vi "main.vi"() -> ()   [LabVIEW 2024]
panel:
  out "Column Names":string[](array[string])
  out "Result Set 3":string[][](table)
  out "?":string[](array[string])
  in  "?":bool
  in  "num_cmd 4":string
  in  "Suppression de la commande":bool
  in  "num_cmd 3":string
  in  "?":bool
  in  "num_cmd 2":string
  in  "date livraison":string
  in  "?":bool
  in  "id produit":string
  in  "nom_produit":string
  in  "date_livraison":string
  in  "date_commande":string
  in  "adresse_client":string
  in  "tele_client":string
  in  "nom_pre_client":string
  in  "status_liv":string
  in  "quantite":string
  in  "description":string
  in  "num_cmd":string
  out "?":string[][](table)
  out "?":string[](array[string])
  out "Result Set 2":string[][](table)
  out "Result Set":string[][](table)
  out "Salaire brut":dbl
  out "Salaire net":dbl
  out "Cout des salaires":dbl
  in  "button calc salaire":bool
  in  "Taux horaire":dbl
  out "notions_cles":dbl[](array[numeric])
  in  "Calculs button":bool
  in  "Impots":dbl
  in  "CA":dbl
  in  "Argent ventes":dbl
  in  "dettes":dbl
  out "Taches":string[][](table) caption="Taches salarié"
  out "Pointages":string[][](table)
  in  "OK Button":bool
  in  "Action":i16(ring) items=["Supprimer un employé", "Ajouter un employé"]
  in  "Choix":i16(ring) items=["admin", "alexis", "julien", "florian", "saco", "aaaaa"]
  in  "Projet":i16(ring) items=["Meuble"]
  out "Taches du projet":string[][](table)
  out "Identifiant de l'employé":string
  out "Code du Poste":dbl
  out "Prénom":string
  out "Nom":string
  out "?":string
  in  "Annuler Licenciement":bool
  in  "Valider Licenciement":bool
  out "?":string
  in  "Annuler Recrutement":bool
  in  "Valider Recrutement":bool
  in  "Mot de passe administrateur":string
  in  "Identifiant de l'employé":string
  in  "Supprimer l'employé":bool
  out "?":string
  in  "Licenciement":bool
  out "?":string
  out "?":string
  in  "Ajouter l'employé":bool
  in  "stop":bool
  in  "Code du Poste":dbl
  in  "Prénom":string
  in  "Nom":string
  in  "Recrutement":bool
  in  "MDP":string
  in  "ID":string
  out "État":string
  in  "Déconnexion":bool
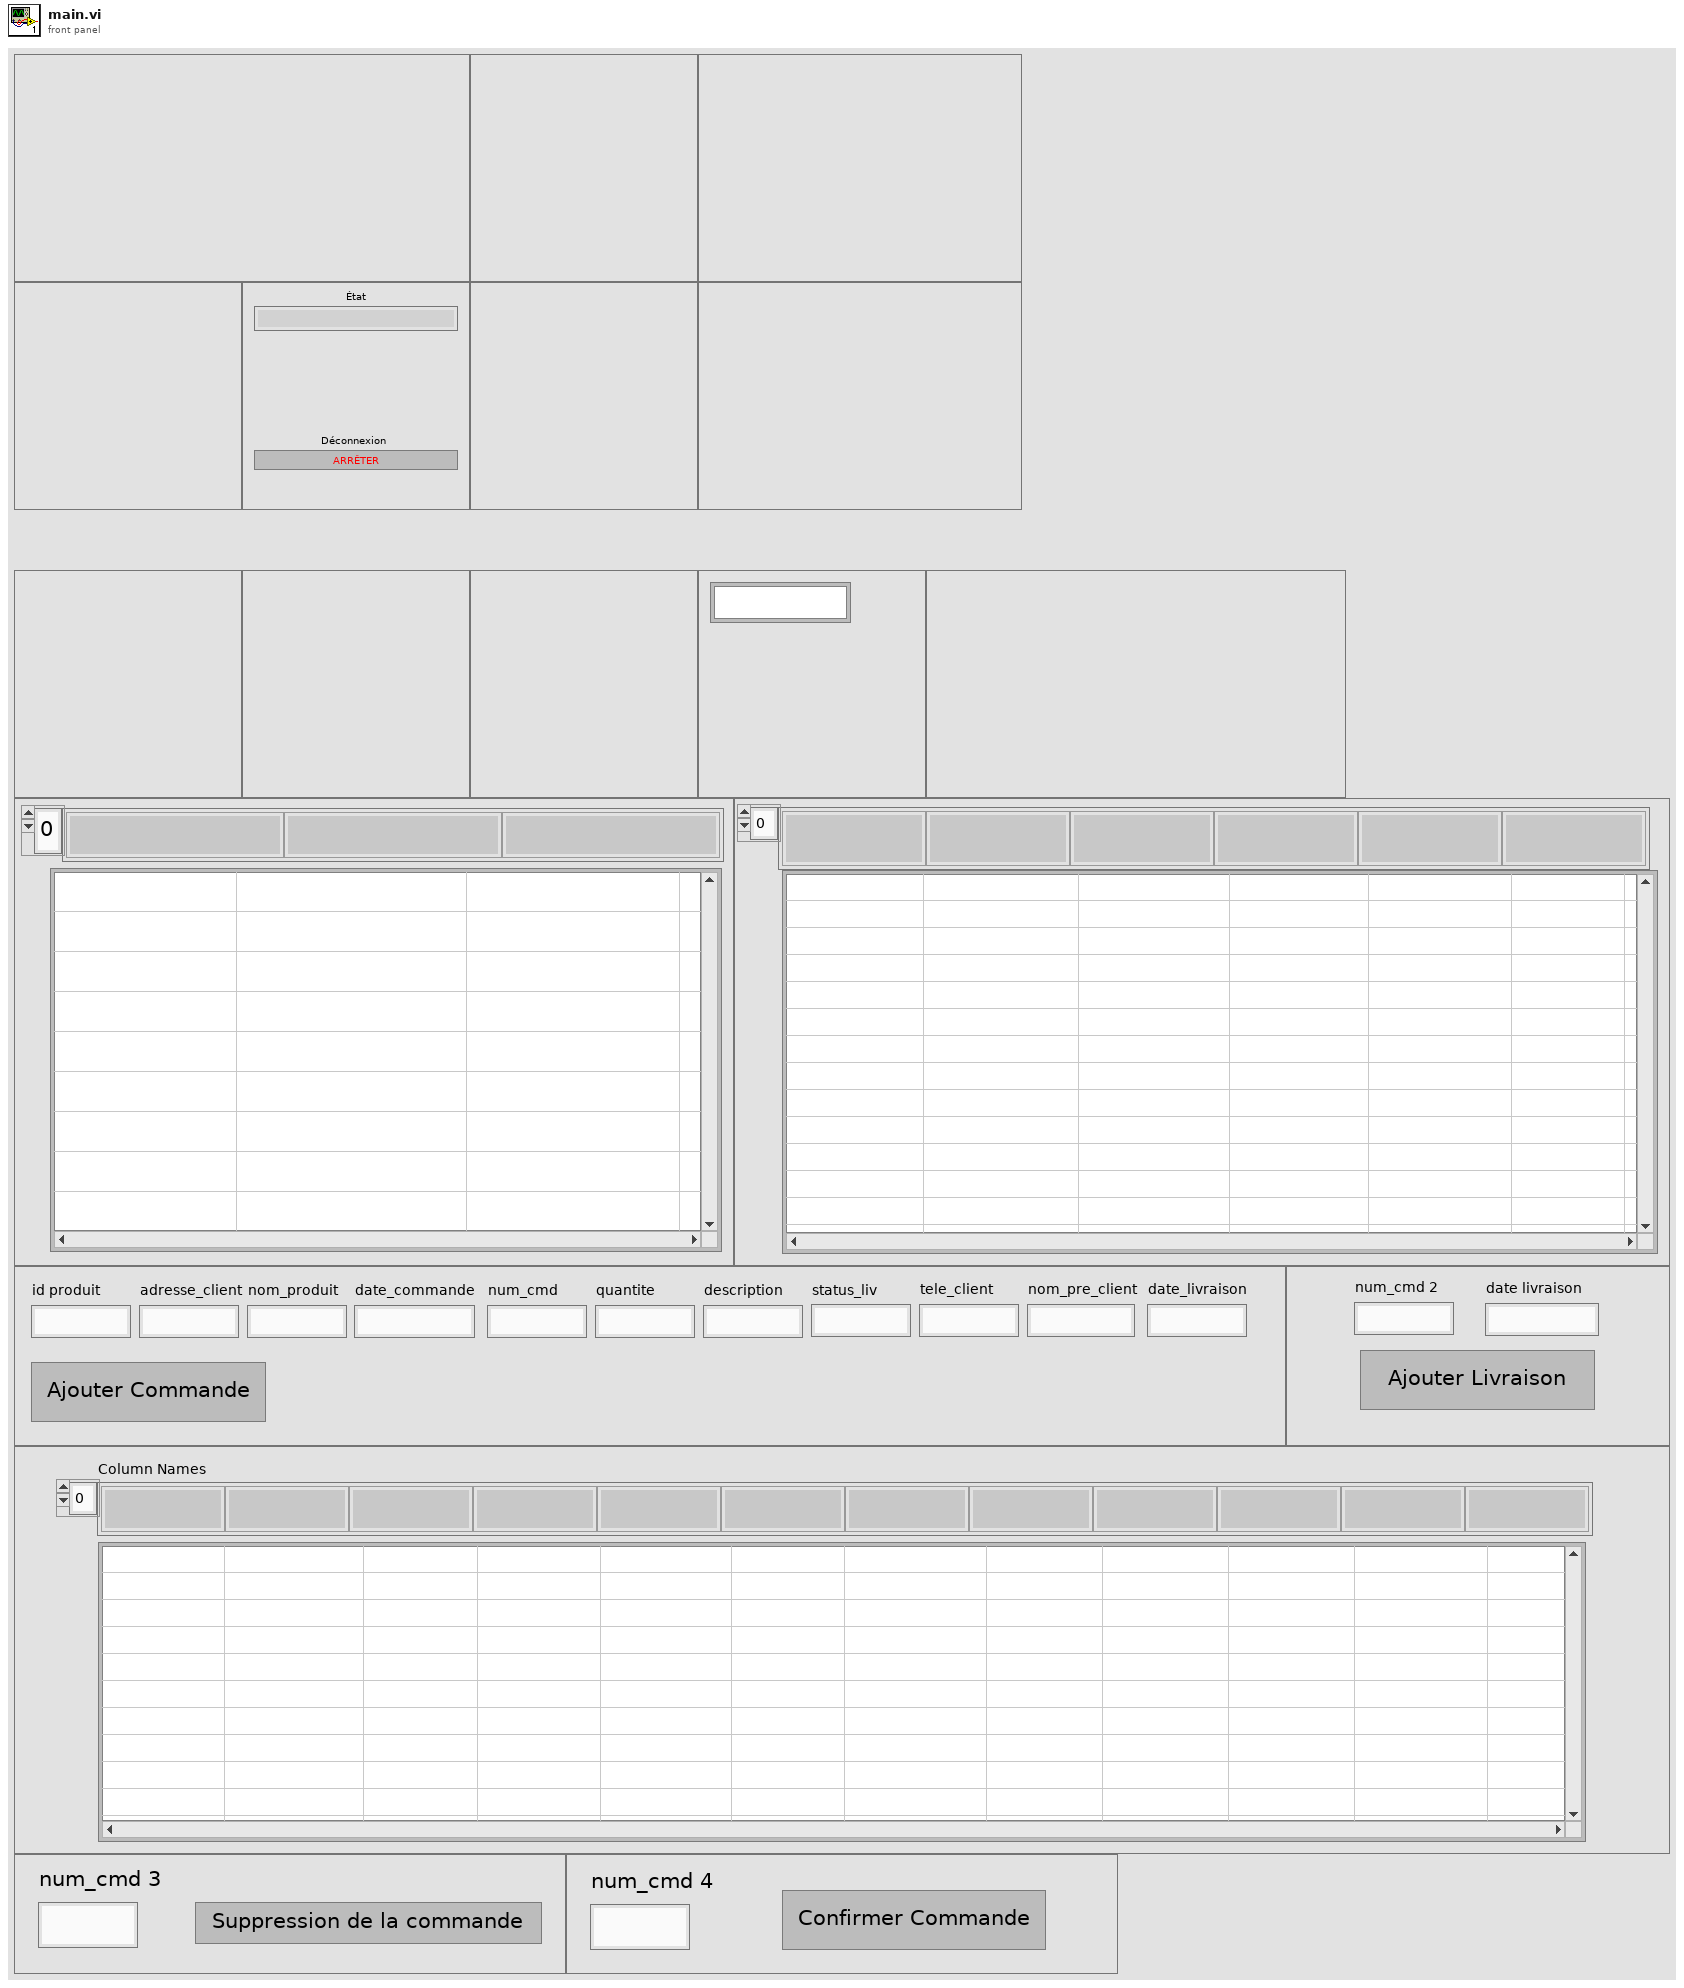
[diagram p1: front panel]
types:
  T1 = enum16{"Gerant", "Ressource Humaine", "Sécurité", "Finance", "Chef de Projet", "Chef de Ligne", "Salarié", "Déconnecter"}
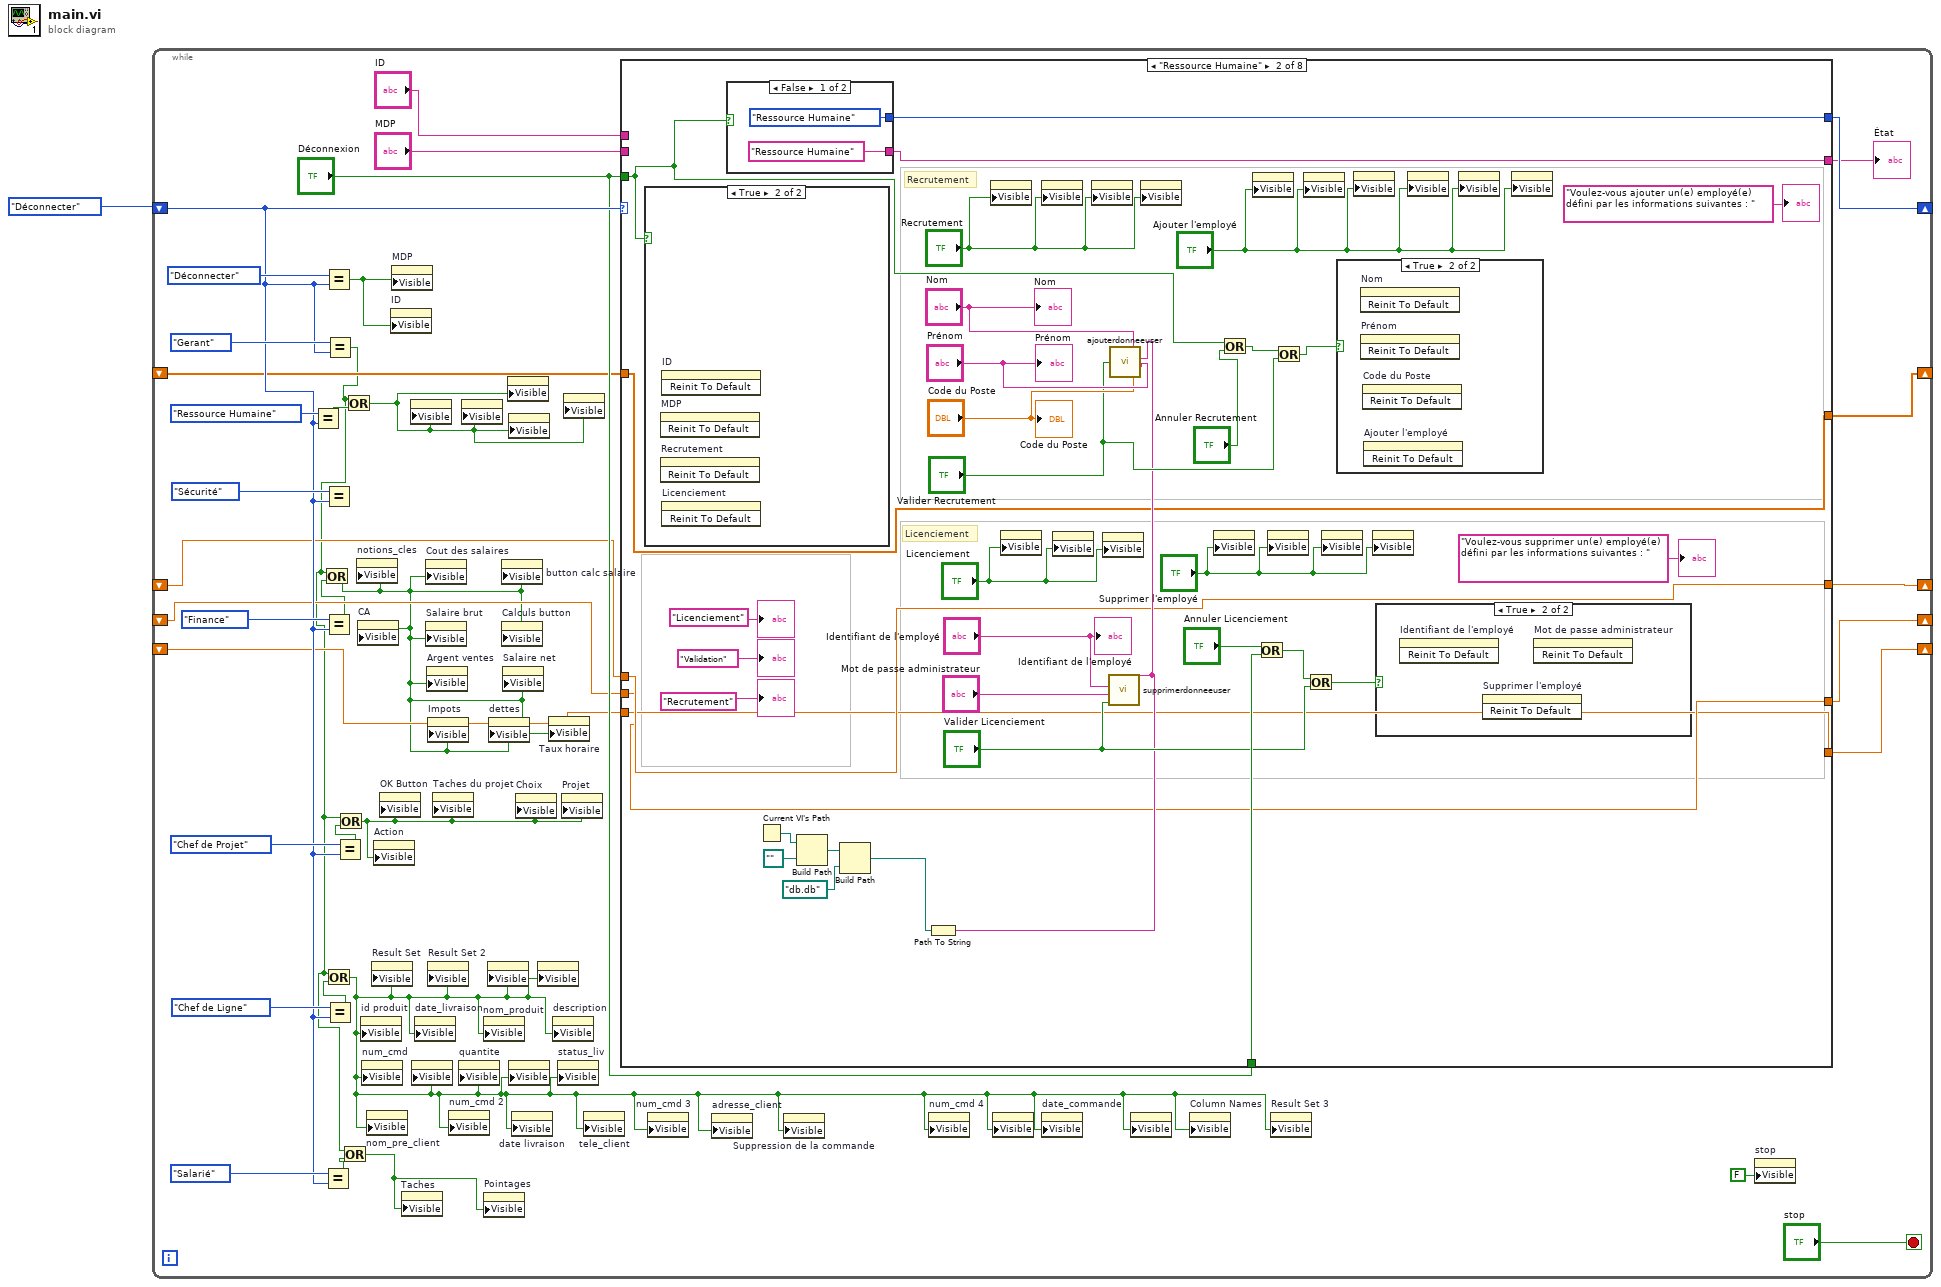
[diagram p0: block diagram]
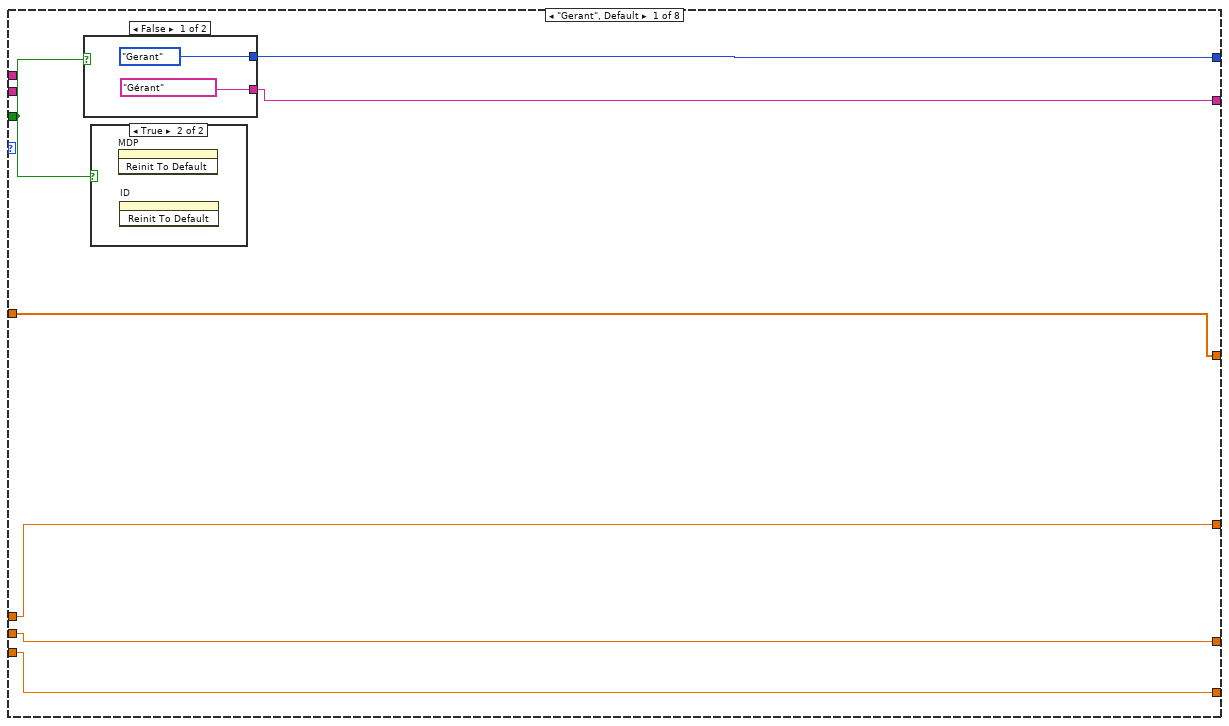
[diagram p2: hidden frame]
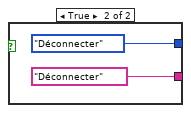
[diagram p4: hidden frame]
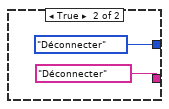
[diagram p8: hidden frame]
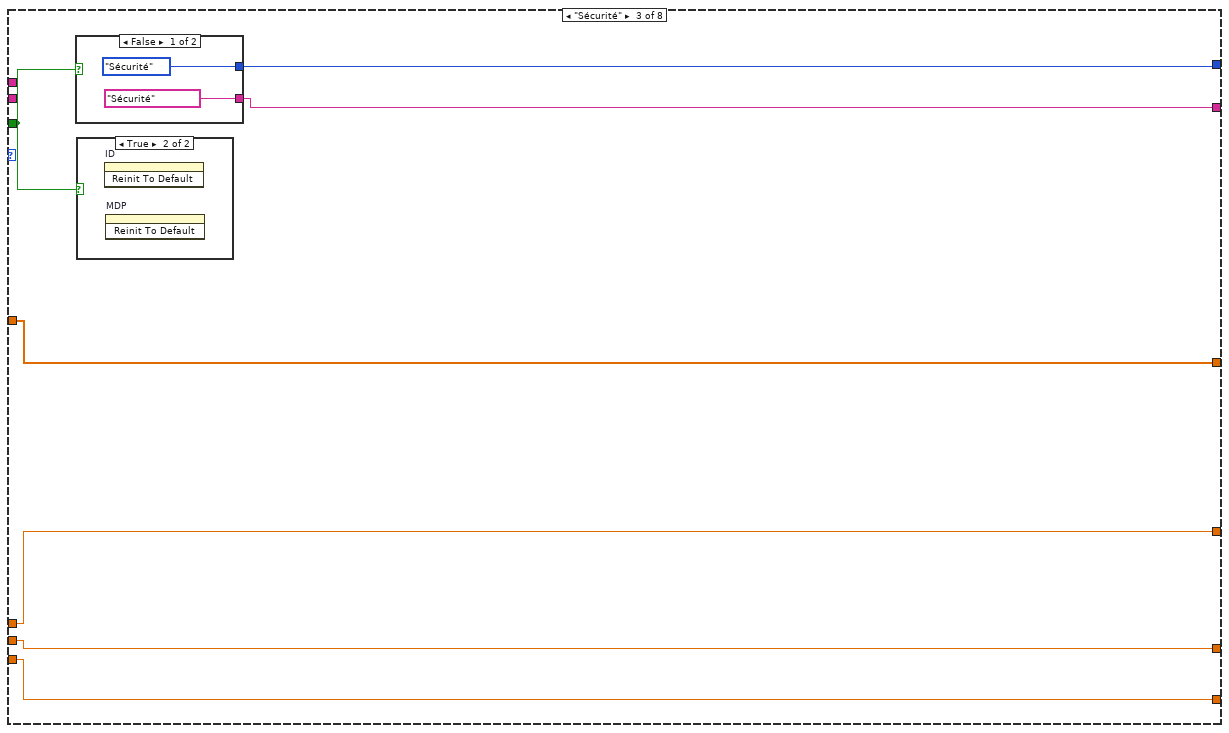
[diagram p9: hidden frame]
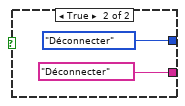
[diagram p11: hidden frame]
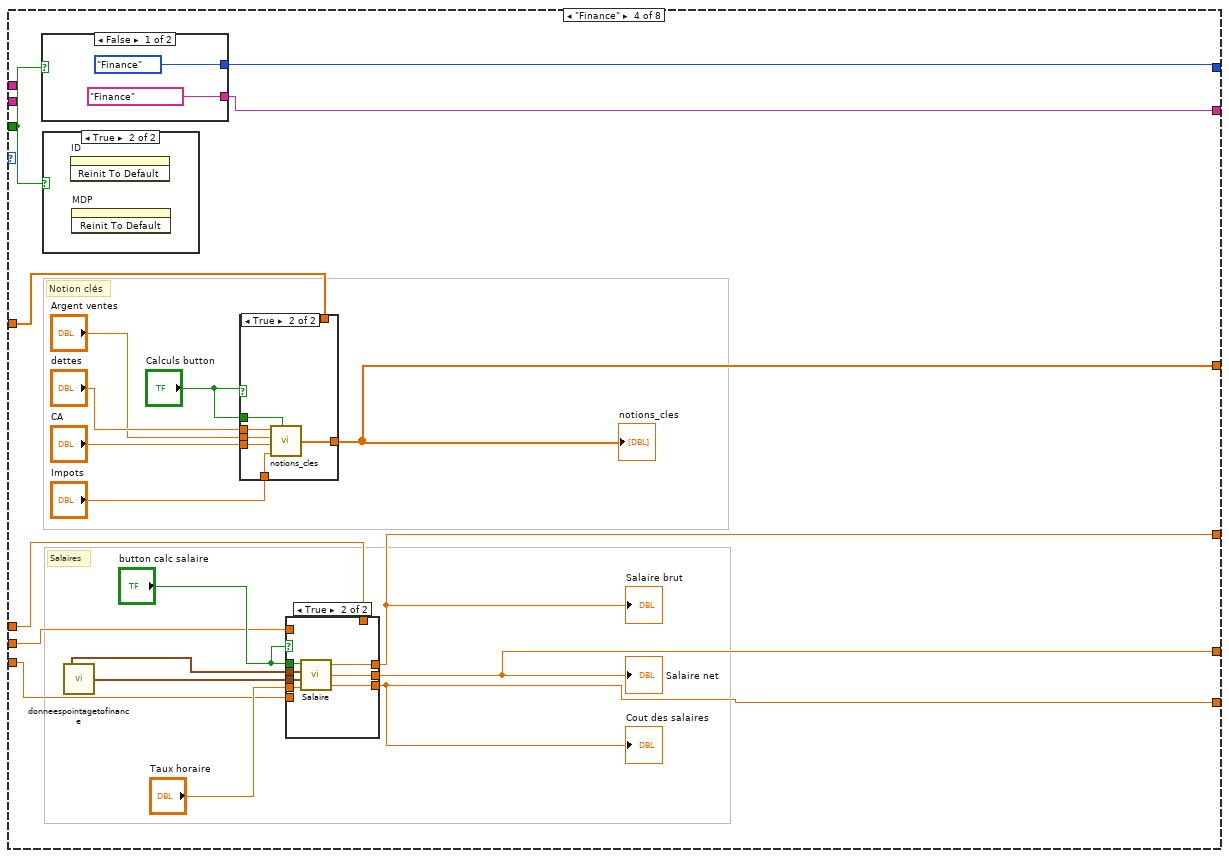
[diagram p12: hidden frame]
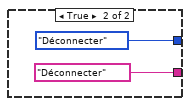
[diagram p16: hidden frame]
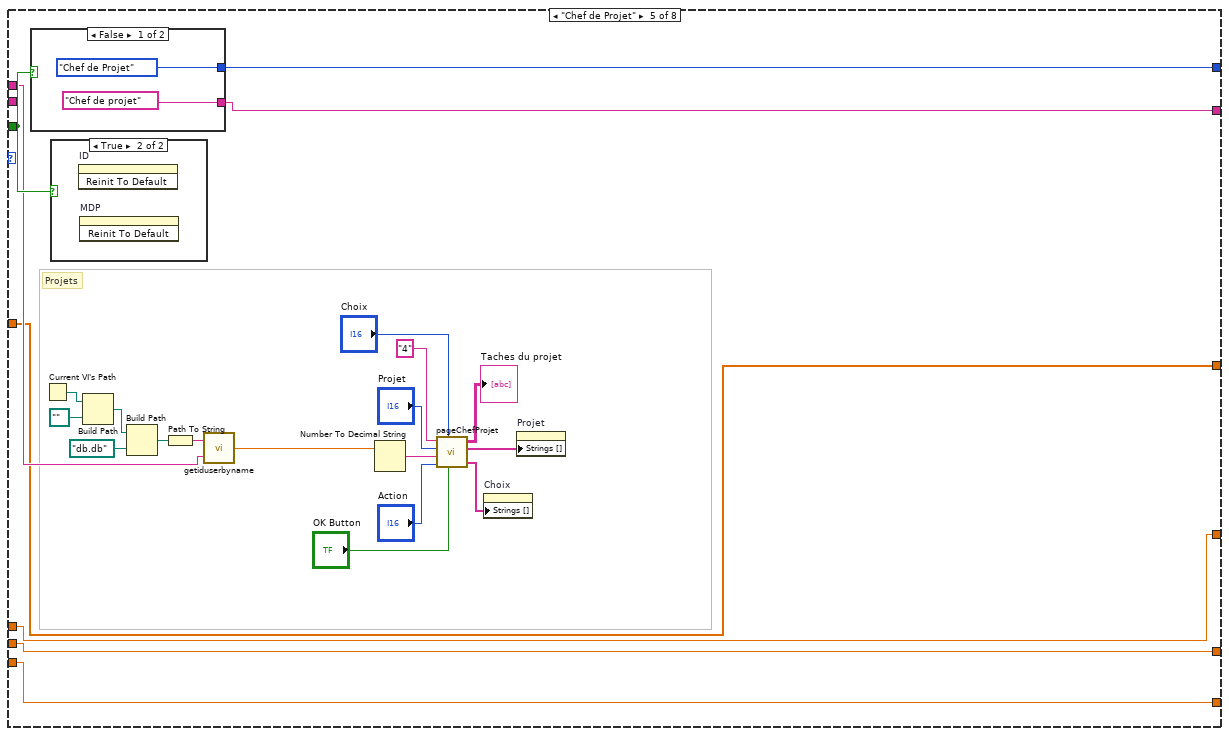
[diagram p17: hidden frame]
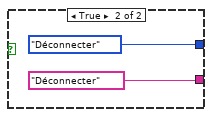
[diagram p19: hidden frame]
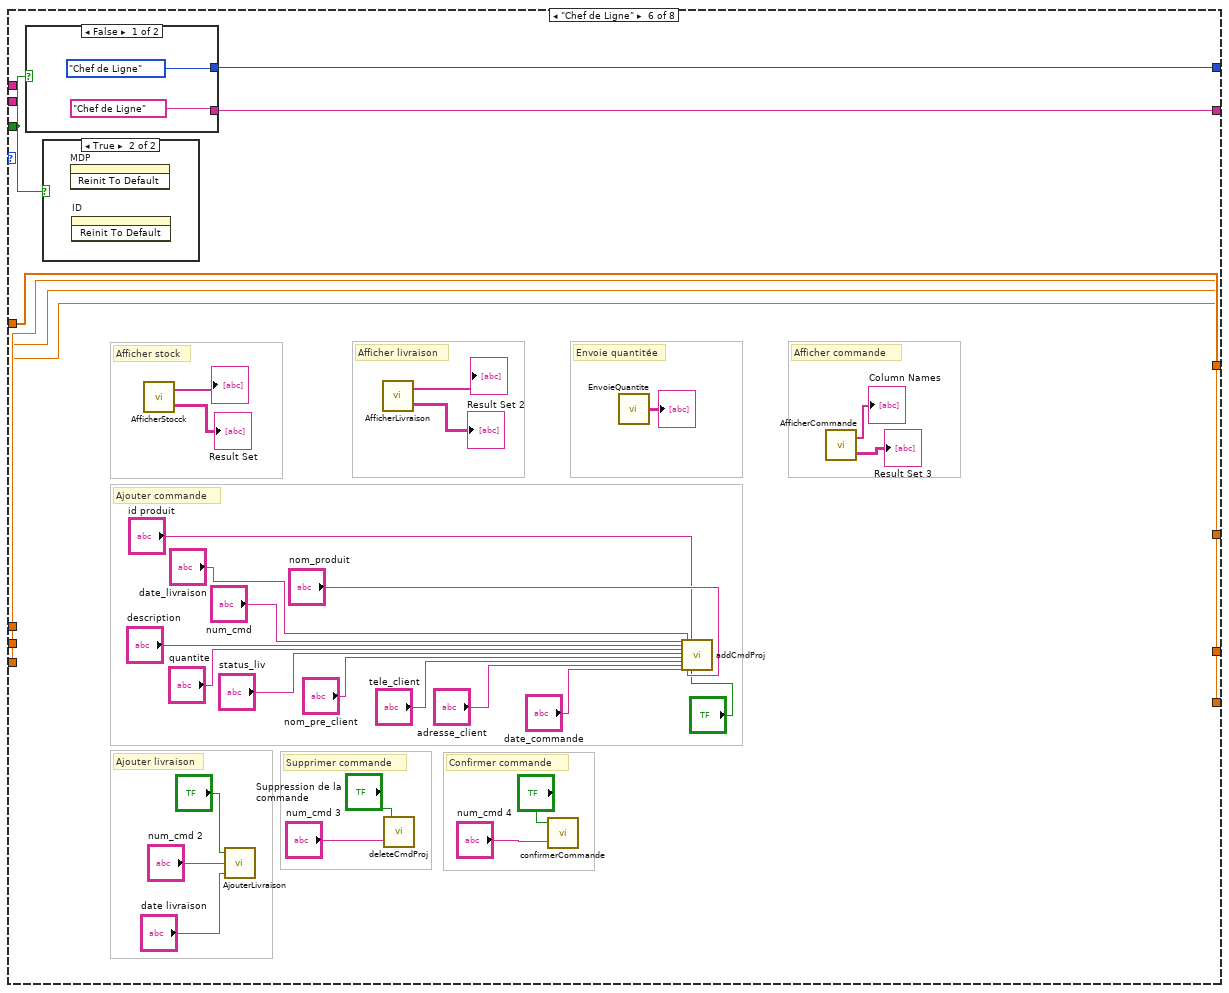
[diagram p20: hidden frame]
diagram:
  n1 = while {
    shift-right: [w37] -> _
    shift-left: T1."Déconnecter" -> [w24]
    shift-right: [w21] -> _
    shift-left: _ -> [w20]
    shift-right: [w18] -> _
    shift-left: _ -> [w19]
    shift-right: [w17] -> _
    shift-left: _ -> [w15]
    shift-right: [w16] -> _
    shift-left: _ -> [w14]
    stop <- "stop" stop-if-true
    n2 = Equal?(x=T1."Ressource Humaine" ("y"), y=w24) -> (x = y?=w11:bool)
    n3 = Equal?(x=T1."Salarié" ("y"), y=w24) -> (x = y?=w4:bool)
    n4 = Equal?(x=T1."Déconnecter" ("y"), y=w24) -> (x = y?=w23:bool)
    n5 = Equal?(x=T1."Sécurité" ("y"), y=w24) -> ()  [unwired: 1 out]
    n6 = Equal?(x=T1."Finance" ("y"), y=w24) -> (x = y?=w9:bool)
    n7 = Equal?(x=T1."Gerant" ("y"), y=w24) -> (x = y?=w3:bool)
    n8 = Or(x=w3, y=w9) -> (x .or. y?=w10:bool)
    n9 = Equal?(x=T1."Chef de Ligne" ("y"), y=w24) -> (x = y?=w6:bool)
    n10 = Or(x=w3, y=w6) -> (x .or. y?=w2:bool)
    n11 = Equal?(x=T1."Chef de Projet" ("y"), y=w24) -> (x = y?=w7:bool)
    n12 = Or(x=w3, y=w7) -> (x .or. y?=w8:bool)
    n13 = Or(x=w3, y=w4) -> (x .or. y?=w5:bool)
    n14 = Or(x=w3, y=w11) -> (x .or. y?=w12:bool)
    n15 = property on="notions_cles" class="Arr (strict)"("Visible"=w10) -> ()  [unwired: 2 in, 2 out]
    n16 = property on="CA" class="DigNum (strict)"("Visible"=w10) -> ()  [unwired: 2 in, 2 out]
    n17 = property on="id produit" class="Str"("Visible"=w2) -> ()  [unwired: 2 in, 2 out]
    n18 = property on="num_cmd" class="Str"("Visible"=w2) -> ()  [unwired: 2 in, 2 out]
    n19 = property on="nom_pre_client" class="Str"("Visible"=w2) -> ()  [unwired: 2 in, 2 out]
    n20 = property on="Result Set" class="Tbl (strict)"("Visible"=w2) -> ()  [unwired: 2 in, 2 out]
    n21 = property on="Action" class="Ring (strict)"("Visible"=w8) -> ()  [unwired: 2 in, 2 out]
    n22 = property on="OK Button" class="Bool"("Visible"=w8) -> ()  [unwired: 2 in, 2 out]
    n23 = property on="ID" class="Str"("Visible"=w23) -> ()  [unwired: 2 in, 2 out]
    n24 = property on="MDP" class="Str"("Visible"=w23) -> ()  [unwired: 2 in, 2 out]
    n25 = property on="Taches" class="Tbl (strict)"("Visible"=w5) -> ()  [unwired: 2 in, 2 out]
    n26 = property on="Recrutement" class="Bool (strict)"("Visible"=w12) -> ()  [unwired: 2 in, 2 out]
    n27 = property class="Bool"("Visible"=w2) -> ()  [unwired: 2 in, 2 out]
    n28 = property on="date_livraison" class="Str"("Visible"=w2) -> ()  [unwired: 2 in, 2 out]
    n29 = property on="Cout des salaires" class="DigNum (strict)"("Visible"=w10) -> ()  [unwired: 2 in, 2 out]
    n30 = property on="Salaire brut" class="DigNum (strict)"("Visible"=w10) -> ()  [unwired: 2 in, 2 out]
    n31 = property on="Argent ventes" class="DigNum (strict)"("Visible"=w10) -> ()  [unwired: 2 in, 2 out]
    n32 = property on="Impots" class="DigNum (strict)"("Visible"=w10) -> ()  [unwired: 2 in, 2 out]
    n33 = property on="Result Set 2" class="Tbl (strict)"("Visible"=w2) -> ()  [unwired: 2 in, 2 out]
    n34 = property on="Taches du projet" class="Tbl (strict)"("Visible"=w8) -> ()  [unwired: 2 in, 2 out]
    n35 = property on="num_cmd 2" class="Str"("Visible"=w2) -> ()  [unwired: 2 in, 2 out]
    n36 = property on="quantite" class="Str"("Visible"=w2) -> ()  [unwired: 2 in, 2 out]
    n37 = property class="Str"("Visible"=w12) -> ()  [unwired: 2 in, 2 out]
    n38 = property on="nom_produit" class="Str"("Visible"=w2) -> ()  [unwired: 2 in, 2 out]
    n39 = property on="Pointages" class="Tbl (strict)"("Visible"=w5) -> ()  [unwired: 2 in, 2 out]
    n40 = property class="Arr (strict)"("Visible"=w2) -> ()  [unwired: 2 in, 2 out]
    n41 = property on="dettes" class="DigNum (strict)"("Visible"=w10) -> ()  [unwired: 2 in, 2 out]
    n42 = property on="button calc salaire" class="Bool"("Visible"=w10) -> ()  [unwired: 2 in, 2 out]
    n43 = property on="Calculs button" class="Bool"("Visible"=w10) -> ()  [unwired: 2 in, 2 out]
    n44 = property on="Salaire net" class="DigNum (strict)"("Visible"=w10) -> ()  [unwired: 2 in, 2 out]
    n45 = property class="Str"("Visible"=w12) -> ()  [unwired: 2 in, 2 out]
    n46 = property on="Licenciement" class="Bool (strict)"("Visible"=w12) -> ()  [unwired: 2 in, 2 out]
    n47 = property class="Bool"("Visible"=w2) -> ()  [unwired: 2 in, 2 out]
    n48 = property on="date livraison" class="Str"("Visible"=w2) -> ()  [unwired: 2 in, 2 out]
    n49 = property on="Choix" class="Ring (strict)"("Visible"=w8) -> ()  [unwired: 2 in, 2 out]
    n50 = property class="Tbl (strict)"("Visible"=w2) -> ()  [unwired: 2 in, 2 out]
    n51 = property on="Taux horaire" class="DigNum (strict)"("Visible"=w10) -> ()  [unwired: 2 in, 2 out]
    n52 = property on="description" class="Str"("Visible"=w2) -> ()  [unwired: 2 in, 2 out]
    n53 = property on="status_liv" class="Str"("Visible"=w2) -> ()  [unwired: 2 in, 2 out]
    n54 = property on="Projet" class="Ring (strict)"("Visible"=w8) -> ()  [unwired: 2 in, 2 out]
    n55 = property class="Str"("Visible"=w12) -> ()  [unwired: 2 in, 2 out]
    n56 = property on="tele_client" class="Str"("Visible"=w2) -> ()  [unwired: 2 in, 2 out]
    n57 = case shown="\"Ressource Humaine\"" w24 {
      tunnel: [w44 w84 w95 w119 w164 w201 w222 w232] -> w37
      tunnel: "Déconnexion" -> [w42 w70 w93 w117 w162 w199 w220 w240]
      tunnel: [w43 w83 w94 w118 w163 w200 w221 w231] -> w36
      tunnel: "ID" -> [_ _ _ _ w160 _ w216 w234]
      tunnel: "MDP" -> [_ _ _ _ _ _ _ w233]
      tunnel: "Déconnexion" -> [_ w72 _ _ _ _ _ _]
      tunnel: [w41 w52 w92 w111 w153 w198 w209 w230] -> w21
      tunnel: w20 -> [w41 w52 w92 w110 w153 w198 w209 w230]
      tunnel: w19 -> [w40 w51 w91 w104 w152 w197 w208 w229]
      tunnel: [w40 w51 w91 w107 w152 w197 w208 w229] -> w18
      tunnel: [w39 w50 w90 w106 w151 w196 w207 w228] -> w17
      tunnel: [w38 w49 w89 w105 w150 w195 w206 w227] -> w16
      tunnel: w15 -> [w39 w50 w90 w103 w151 w196 w207 w228]
      tunnel: w14 -> [w38 w49 w89 w102 w150 w195 w206 w227]
      frame "Gerant", Default {
        n58 = case shown="False" w42 {
          tunnel: [T1."Gerant" T1."Déconnecter"] -> w44
          tunnel: ["Gérant" "Déconnecter"] -> w43
          frame False {
          }
          frame True {
          }
        }
        n59 = case shown="True" w42 {
          frame False {
          }
          frame True {
            n60 = invoke on="MDP" class="Ch" method="Reinit To Default"() -> ()  [unwired: 3 in, 3 out]
            n61 = invoke on="ID" class="Ch" method="Reinit To Default"() -> ()  [unwired: 3 in, 3 out]
          }
        }
      }
      frame "Ressource Humaine" {
        # "Licenciement"
        # "Recrutement"
        n62 = case shown="True" w70 {
          frame False {
          }
          frame True {
            n63 = invoke on="MDP" class="Ch" method="Reinit To Default"() -> ()  [unwired: 3 in, 3 out]
            n64 = invoke on="Recrutement" class="Bool (strict)" method="Reinit To Default"() -> ()  [unwired: 3 in, 3 out]
            n65 = invoke on="ID" class="Ch" method="Reinit To Default"() -> ()  [unwired: 3 in, 3 out]
            n66 = invoke on="Licenciement" class="Bool (strict)" method="Reinit To Default"() -> ()  [unwired: 3 in, 3 out]
          }
        }
        n67 = case shown="False" w70 {
          tunnel: [T1."Ressource Humaine" T1."Déconnecter"] -> w84
          tunnel: ["Ressource Humaine" "Déconnecter"] -> w83
          frame False {
          }
          frame True {
          }
        }
        n68 = Current VI's Path() -> (path=w58:path)
        n69 = Build Path(base path=w58, name or relative path=path "..") -> (appended path=w55:path)
        n70 = Build Path(base path=w55, name or relative path=path "db.db" ("Filename")) -> (appended path=w54:path)
        n71 = Path To String(path=w54) -> (string=w53:string)
        n72 = property on="Code du Poste" class="DigNum (strict)"("Visible"="Recrutement") -> ()  [unwired: 2 in, 2 out]
        n73 = property on="Identifiant de l'employé" class="Str"("Visible"="Licenciement") -> ()  [unwired: 2 in, 2 out]
        n74 = property on="Nom" class="Str"("Visible"="Recrutement") -> ()  [unwired: 2 in, 2 out]
        n75 = property on="Mot de passe administrateur" class="Str"("Visible"="Licenciement") -> ()  [unwired: 2 in, 2 out]
        n76 = property on="Prénom" class="Str"("Visible"="Recrutement") -> ()  [unwired: 2 in, 2 out]
        n77 = property on="Supprimer l'employé" class="Bool (strict)"("Visible"="Licenciement") -> ()  [unwired: 2 in, 2 out]
        n78 = call "supprimerdonneeuser.vi"("Validation"="Valider Licenciement", "AdminPassword"="Mot de passe administrateur", "Identifiant"="Identifiant de l'employé", "Fichier DB"=w53) -> ()
        n79 = call "ajouterdonneeuser.vi"("Validation"="Valider Recrutement", "Nom"="Nom", "Fichier DB"=w53, "Prénom"="Prénom", "Code du poste"="Code du Poste") -> ()
        n80 = property on="Ajouter l'employé" class="Bool (strict)"("Visible"="Recrutement") -> ()  [unwired: 2 in, 2 out]
        n81 = property class="Str"("Visible"="Supprimer l'employé") -> ()  [unwired: 2 in, 2 out]
        n82 = Or(x=w70, y="Annuler Recrutement") -> (x .or. y?=w63:bool)
        n83 = property on="Valider Recrutement" class="Bool"("Visible"="Ajouter l'employé") -> ()  [unwired: 2 in, 2 out]
        n84 = Or(x="Annuler Licenciement", y=w72) -> (x .or. y?=w60:bool)
        n85 = property on="Valider Licenciement" class="Bool"("Visible"="Supprimer l'employé") -> ()  [unwired: 2 in, 2 out]
        n86 = Or(x=w63, y="Valider Recrutement") -> (x .or. y?=w62:bool)
        n87 = property on="Annuler Recrutement" class="Bool"("Visible"="Ajouter l'employé") -> ()  [unwired: 2 in, 2 out]
        n88 = Or(x=w60, y="Valider Licenciement") -> (x .or. y?=w59:bool)
        n89 = property on="Annuler Licenciement" class="Bool"("Visible"="Supprimer l'employé") -> ()  [unwired: 2 in, 2 out]
        n90 = case shown="True" w62 {
          frame False {
          }
          frame True {
            n91 = invoke on="Nom" class="Ch" method="Reinit To Default"() -> ()  [unwired: 3 in, 3 out]
            n92 = invoke on="Prénom" class="Ch" method="Reinit To Default"() -> ()  [unwired: 3 in, 3 out]
            n93 = invoke on="Code du Poste" class="NumNb (strict)" method="Reinit To Default"() -> ()  [unwired: 3 in, 3 out]
            n94 = invoke on="Ajouter l'employé" class="Bool (strict)" method="Reinit To Default"() -> ()  [unwired: 3 in, 3 out]
          }
        }
        n95 = property class="Str"("Visible"="Ajouter l'employé") -> ()  [unwired: 2 in, 2 out]
        n96 = property on="Identifiant de l'employé" class="Str"("Visible"="Supprimer l'employé") -> ()  [unwired: 2 in, 2 out]
        n97 = case shown="True" w59 {
          frame False {
          }
          frame True {
            n98 = invoke on="Identifiant de l'employé" class="Ch" method="Reinit To Default"() -> ()  [unwired: 3 in, 3 out]
            n99 = invoke on="Supprimer l'employé" class="Bool (strict)" method="Reinit To Default"() -> ()  [unwired: 3 in, 3 out]
            n100 = invoke on="Mot de passe administrateur" class="Ch" method="Reinit To Default"() -> ()  [unwired: 3 in, 3 out]
          }
        }
        n101 = property on="Nom" class="Str"("Visible"="Ajouter l'employé") -> ()  [unwired: 2 in, 2 out]
        n102 = property on="Prénom" class="Str"("Visible"="Ajouter l'employé") -> ()  [unwired: 2 in, 2 out]
        n103 = property on="Code du Poste" class="DigNum (strict)"("Visible"="Ajouter l'employé") -> ()  [unwired: 2 in, 2 out]
        "?" <- "Validation"
        "?" <- "Licenciement"
        "?" <- "Recrutement"
        "?" <- "Voulez-vous ajouter un(e) employé(e) défini par les informations suivantes : "
        "?" <- "Voulez-vous supprimer un(e) employé(e) défini par les informations suivantes : "
        "Nom" <- "Nom"
        "Prénom" <- "Prénom"
        "Code du Poste" <- "Code du Poste"
        "Identifiant de l'employé" <- "Identifiant de l'employé"
      }
      frame "Sécurité" {
        n104 = case shown="False" w93 {
          tunnel: [T1."Sécurité" T1."Déconnecter"] -> w95
          tunnel: ["Sécurité" "Déconnecter"] -> w94
          frame False {
          }
          frame True {
          }
        }
        n105 = case shown="True" w93 {
          frame False {
          }
          frame True {
            n106 = invoke on="ID" class="Ch" method="Reinit To Default"() -> ()  [unwired: 3 in, 3 out]
            n107 = invoke on="MDP" class="Ch" method="Reinit To Default"() -> ()  [unwired: 3 in, 3 out]
          }
        }
      }
      frame "Finance" {
        # "Salaires"
        # "Notion clés"
        n108 = case shown="False" w117 {
          tunnel: [T1."Finance" T1."Déconnecter"] -> w119
          tunnel: ["Finance" "Déconnecter"] -> w118
          frame False {
          }
          frame True {
          }
        }
        n109 = case shown="True" w117 {
          frame False {
          }
          frame True {
            n110 = invoke on="ID" class="Ch" method="Reinit To Default"() -> ()  [unwired: 3 in, 3 out]
            n111 = invoke on="MDP" class="Ch" method="Reinit To Default"() -> ()  [unwired: 3 in, 3 out]
          }
        }
        n112 = call "donneespointagetofinance.vi"() -> ("Date_fin"=w100:timestamp[], "Date_debut"=w101:timestamp[])
        n113 = case shown="True" "Calculs button" {
          tunnel: "dettes" -> [_ w136]
          tunnel: "Argent ventes" -> [_ w135]
          tunnel: "CA" -> [_ w134]
          tunnel: "Impots" -> [_ w133]
          tunnel: "Calculs button" -> [_ w132]
          tunnel: [w130 w131] -> w111
          tunnel: w110 -> [w130 _]
          frame False {
          }
          frame True {
            n114 = call "notions_cles.vi"("dettes"=w136, "Argent ventes"=w135, "CA"=w134, "Impots"=w133, "Calculs button"=w132) -> ("notions_cles"=w131:dbl[])
          }
        }
        "notions_cles" <- w111
        n115 = case shown="True" "button calc salaire" {
          tunnel: "Taux horaire" -> [_ w129]
          tunnel: w100 -> [_ w128]
          tunnel: w101 -> [_ w127]
          tunnel: "button calc salaire" -> [_ w126]
          tunnel: [w120 w125] -> w105
          tunnel: [w121 w124] -> w106
          tunnel: [w122 w123] -> w107
          tunnel: w104 -> [w122 _]
          tunnel: w103 -> [w121 _]
          tunnel: w102 -> [w120 _]
          frame False {
          }
          frame True {
            n116 = call "Salaire.vi"("Taux horaire"=w129, "Tableau heures fin employé"=w128, "Tableau heures debut employé"=w127, "button calc salaire"=w126) -> ("Cout des salaires"=w125:dbl, "Salaire net"=w124:dbl, "Salaire brut"=w123:dbl)
          }
        }
        "Cout des salaires" <- w105
        "Salaire net" <- w106
        "Salaire brut" <- w107
      }
      frame "Chef de Projet" {
        # "Projets"
        n117 = case shown="False" w162 {
          tunnel: [T1."Chef de Projet" T1."Déconnecter"] -> w164
          tunnel: ["Chef de projet" "Déconnecter"] -> w163
          frame False {
          }
          frame True {
          }
        }
        n118 = Current VI's Path() -> (path=w159:path)
        n119 = case shown="True" w162 {
          frame False {
          }
          frame True {
            n120 = invoke on="ID" class="Ch" method="Reinit To Default"() -> ()  [unwired: 3 in, 3 out]
            n121 = invoke on="MDP" class="Ch" method="Reinit To Default"() -> ()  [unwired: 3 in, 3 out]
          }
        }
        n122 = Build Path(base path=w159, name or relative path=path "..") -> (appended path=w156:path)
        n123 = Build Path(base path=w156, name or relative path=path "db.db" ("Filename")) -> (appended path=w154:path)
        n124 = Path To String(path=w154) -> (string=w155:string)
        n125 = call "getiduserbyname.vi"("name"=w160, "Fichier DB"=w155) -> ("id"=w161:dbl)
        n126 = Number To Decimal String(number=w161) -> (decimal integer string=w149:string)  [unwired: 1 in]
        n127 = call "pageChefProjet.vi"("role"="4", "Choix"="Choix", "Projet"="Projet", "id_personnel_connect"=w149, "OK Button"="OK Button", "Action"="Action") -> ("Table Control"=→"Taches du projet":string[][], "liste_projet"=w142:string[], "liste_personnel"=w141:string[])
        n128 = property on="Choix" class="Ring (strict)"("Strings []"=w141) -> ()  [unwired: 2 in, 2 out]
        n129 = property on="Projet" class="Ring (strict)"("Strings []"=w142) -> ()  [unwired: 2 in, 2 out]
      }
      frame "Chef de Ligne" {
        # "Afficher commande"
        # "Confirmer commande"
        # "Supprimer commande"
        # "Ajouter livraison"
        # "Ajouter commande"
        # "Envoie quantitée"
        # "Afficher livraison"
        # "Afficher stock"
        n130 = case shown="False" w199 {
          tunnel: [T1."Chef de Ligne" T1."Déconnecter"] -> w201
          tunnel: ["Chef de Ligne" "Déconnecter"] -> w200
          frame False {
          }
          frame True {
          }
        }
        n131 = case shown="True" w199 {
          frame False {
          }
          frame True {
            n132 = invoke on="MDP" class="Ch" method="Reinit To Default"() -> ()  [unwired: 3 in, 3 out]
            n133 = invoke on="ID" class="Ch" method="Reinit To Default"() -> ()  [unwired: 3 in, 3 out]
          }
        }
        n134 = call "AfficherStocck.vi"() -> ("Result Set"=→"Result Set":string[][], 1:→"?":string[])  [unwired: 2 in]
        n135 = call "AjouterLivraison.vi"("date livraison"="date livraison", "num_cmd"="num_cmd 2", 3:"?") -> ()  [unwired: 1 in]
        n136 = call "AfficherLivraison.vi"() -> ("Result Set"=→"Result Set 2":string[][], 1:→"?":string[])  [unwired: 2 in]
        n137 = call "deleteCmdProj.vi"("num_cmd"="num_cmd 3", "Suppression de la commande"="Suppression de la commande") -> ()  [unwired: 1 in]
        n138 = call "confirmerCommande.vi"("num_cmd"="num_cmd 4", 2:"?") -> ()  [unwired: 1 in]
        n139 = call "EnvoieQuantite.vi"() -> (0:→"?":string[][])  [unwired: 1 in]
        n140 = call "addCmdProj.vi"("num_cmd"="num_cmd", "description"="description", "quantite"="quantite", "status_liv"="status_liv", "nom_pre_client"="nom_pre_client", "tele_client"="tele_client", "adresse_client"="adresse_client", "date_commande"="date_commande", "date_livraison"="date_livraison", "nom_produit"="nom_produit", "id produit"="id produit", 11:"?") -> ()  [unwired: 16 in]
        n141 = call "AfficherCommande.vi"() -> ("Result Set"=→"Result Set 3":string[][], "Column Names"=→"Column Names":string[])  [unwired: 2 in]
      }
      frame "Salarié" {
        # "Projets"
        n142 = case shown="False" w220 {
          tunnel: [T1."Salarié" T1."Déconnecter"] -> w222
          tunnel: ["Salarié" "Déconnecter"] -> w221
          frame False {
          }
          frame True {
          }
        }
        n143 = case shown="True" w220 {
          frame False {
          }
          frame True {
            n144 = invoke on="ID" class="Ch" method="Reinit To Default"() -> ()  [unwired: 3 in, 3 out]
            n145 = invoke on="MDP" class="Ch" method="Reinit To Default"() -> ()  [unwired: 3 in, 3 out]
          }
        }
        n146 = Current VI's Path() -> (path=w215:path)
        n147 = Build Path(base path=w215, name or relative path=path "..") -> (appended path=w212:path)
        n148 = Build Path(base path=w212, name or relative path=path "db.db" ("Filename")) -> (appended path=w211:path)
        n149 = Path To String(path=w211) -> (string=w210:string)
        n150 = call "getiduserbyname.vi"("name"=w216, "Fichier DB"=w210) -> ("id"=w217:dbl)
        n151 = call "getdonneestacheuser.vi"("id"=w217, "Fichier DB"=w210) -> ("Données tache user"=→"Taches":string[][])
        n152 = call "getpointagebyuserid.vi"("id"=w217, "Fichier DB"=w210) -> ("Données pointage"=→"Pointages":string[][])
      }
      frame "Déconnecter" {
        w237 = FALSE ("Visible")
        w238 = FALSE ("Visible")
        w239 = FALSE ("Visible")
        w236 = FALSE ("Visible")
        # "Ressource humaine"
        n153 = property class="Str"("Visible"=w237) -> ()  [unwired: 2 in, 2 out]
        n154 = property on="Identifiant de l'employé" class="Str"("Visible"=w238) -> ()  [unwired: 2 in, 2 out]
        n155 = property on="Nom" class="Str"("Visible"=w236) -> ()  [unwired: 2 in, 2 out]
        n156 = property on="Nom" class="Str"("Visible"=w239) -> ()  [unwired: 2 in, 2 out]
        n157 = call "identification.vi"("Password"=w233, "Identifiant"=w234) -> ("role"=w235:string)  [unwired: 1 out]
        n158 = property on="Annuler Licenciement" class="Bool"("Visible"=w237) -> ()  [unwired: 2 in, 2 out]
        n159 = property on="Mot de passe administrateur" class="Str"("Visible"=w238) -> ()  [unwired: 2 in, 2 out]
        n160 = property on="Prénom" class="Str"("Visible"=w239) -> ()  [unwired: 2 in, 2 out]
        n161 = property on="Prénom" class="Str"("Visible"=w236) -> ()  [unwired: 2 in, 2 out]
        n162 = case shown="\"2\"" w235 {
          tunnel: [T1."Gerant" T1."Ressource Humaine" T1."Sécurité" T1."Finance" T1."Chef de Projet" T1."Chef de Ligne" T1."Salarié" T1."Déconnecter"] -> w232
          tunnel: ["Gérant" "Ressource Humaine" "Gérant" "Gérant" "Gérant" "Gérant" "Gérant" "Déconnecter"] -> w231
          frame "0" {
          }
          frame "1" {
          }
          frame "2" {
          }
          frame "3" {
          }
          frame "4" {
          }
          frame "5" {
          }
          frame "6" {
          }
          frame "7", Default {
          }
        }
        n163 = property on="Supprimer l'employé" class="Bool (strict)"("Visible"=w238) -> ()  [unwired: 2 in, 2 out]
        n164 = property on="Valider Licenciement" class="Bool"("Visible"=w237) -> ()  [unwired: 2 in, 2 out]
        n165 = case shown="True" w240 {
          frame False {
          }
          frame True {
            n166 = invoke on="ID" class="Ch" method="Reinit To Default"() -> ()  [unwired: 3 in, 3 out]
            n167 = invoke on="MDP" class="Ch" method="Reinit To Default"() -> ()  [unwired: 3 in, 3 out]
          }
        }
        n168 = property on="Code du Poste" class="DigNum (strict)"("Visible"=w239) -> ()  [unwired: 2 in, 2 out]
        n169 = property on="Annuler Recrutement" class="Bool"("Visible"=w236) -> ()  [unwired: 2 in, 2 out]
        n170 = property on="Ajouter l'employé" class="Bool (strict)"("Visible"=w239) -> ()  [unwired: 2 in, 2 out]
        n171 = property on="Identifiant de l'employé" class="Str"("Visible"=w237) -> ()  [unwired: 2 in, 2 out]
        n172 = property on="Valider Recrutement" class="Bool"("Visible"=w236) -> ()  [unwired: 2 in, 2 out]
        n173 = property on="Code du Poste" class="DigNum (strict)"("Visible"=w236) -> ()  [unwired: 2 in, 2 out]
        n174 = property class="Str"("Visible"=w236) -> ()  [unwired: 2 in, 2 out]
      }
    }
    "État" <- w36
    n175 = property on="num_cmd 3" class="Str"("Visible"=w2) -> ()  [unwired: 2 in, 2 out]
    n176 = property on="adresse_client" class="Str"("Visible"=w2) -> ()  [unwired: 2 in, 2 out]
    n177 = property on="Suppression de la commande" class="Bool"("Visible"=w2) -> ()  [unwired: 2 in, 2 out]
    n178 = property on="num_cmd 4" class="Str"("Visible"=w2) -> ()  [unwired: 2 in, 2 out]
    n179 = property class="Bool"("Visible"=w2) -> ()  [unwired: 2 in, 2 out]
    n180 = property on="date_commande" class="Str"("Visible"=w2) -> ()  [unwired: 2 in, 2 out]
    n181 = property class="Arr (strict)"("Visible"=w2) -> ()  [unwired: 2 in, 2 out]
    n182 = property on="Column Names" class="Arr (strict)"("Visible"=w2) -> ()  [unwired: 2 in, 2 out]
    n183 = property on="Result Set 3" class="Tbl (strict)"("Visible"=w2) -> ()  [unwired: 2 in, 2 out]
    n184 = property on="stop" class="Bool"("Visible"=FALSE) -> ()  [unwired: 2 in, 2 out]
  }
